vi "PH_gentec_Powermeter.Close.vi"(1 "Connection in":T1, 2 "Device Error in":errorcluster, 3 "Error Message":string, 4 "VISA Refnum in":refnum<visa-resource-name>) -> (0 "Connection out":T1)   [LabVIEW 2014, in "PH_gentec_Powermeter.lvlib"]
uses:
  PH_gentec_Powermeter.lvlib
  PH_Basics/PH_Powermeter_BaseClass/PH_Powermeter_BaseClass.Connection.ctl
  PH_Basics/PH_Powermeter_BaseClass/PH_Powermeter_BaseClass.State.ctl
  instr.lib/gentec-SOLO-PE/gentec-SOLO-PE - Driver.lvlib
  PH_Basics/PH_Powermeter_BaseClass/PH_Powermeter_BaseClass.lvlib
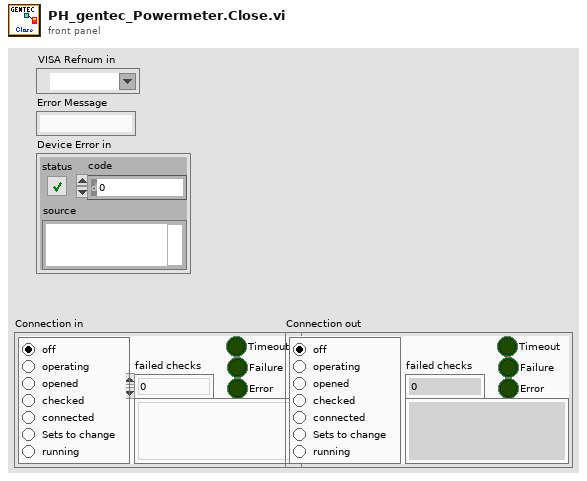
[diagram p1: front panel]
types:
  T1 = typedef "PH_Powermeter_BaseClass.lvlib/PH_Powermeter_BaseClass.Connection.ctl" = cluster{"failed checks":i8, "Timeout":bool, "Data read":string, "Failure":bool, "Error":bool, "State":T2}
  T2 = typedef "PH_Powermeter_BaseClass.lvlib/PH_Powermeter_BaseClass.State.ctl" = enum32{"off", "operating", "opened", "checked", "connected", "Sets to change", "running"}
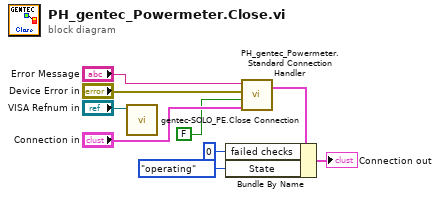
[diagram p0: block diagram]
diagram:
  n1 = call "gentec-SOLO_PE.Close Connection.vi"("VISA resource name in"="VISA Refnum in") -> ()  [unwired: 6 in, 1 out]
  n2 = call "PH_gentec_Powermeter.Standard Connection Handler.vi"("Connection in"="Connection in", "Timeout"=FALSE ("opened"), "Device Error"="Device Error in", "Error"="Error Message") -> ("Connection out"=w6:T1)  [unwired: 1 out]
  n3 = Bundle By Name(cluster=w6, "failed checks"=i8 0, "State"=PH_Powermeter_BaseClass.State."operating") -> (→"Connection out":T1)
